vi "Change_RunInfo_V2.vi"(2 "error in (no error)":errorcluster, 3 "Run Data SubPanel in":T1) -> (0 "error out":errorcluster, 1 "Run Data SubPanel out":T1)   [LabVIEW 2019]
uses:
  Controls/DataBlockControl.ctl
panel:
  in  "Change Test Type":bool
  in  "Effective LET":bool
  in  "Update Board Number":bool
  in  "Update Ion":bool
  in  "Update DUT":bool
  in  "Update Path":bool
  out "Current Run Data":T1
  in  "Exit SubVI":bool
  in  "Run Data Input":T1
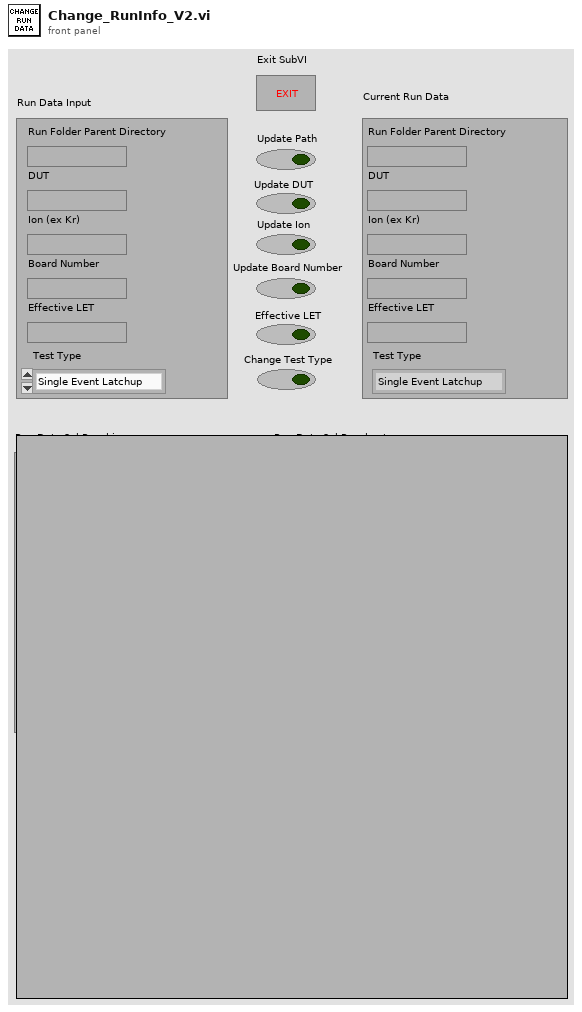
[diagram p1: front panel]
types:
  T1 = typedef "DataBlockControl.ctl" = cluster{"Run Folder Parent Directory":path, "DUT":string, "Ion (ex Kr)":string, "Board Number":string, "Effective LET":string, "Test Type":enum16{"Single Event Latchup", "Single Event Transient", "Single Event Upset"}}
  T2 = enum16{"Single Event Latchup", "Single Event Transient", "Single Event Upset"}
  T3 = cluster{"Run Folder Parent Directory":path, "DUT":string, "Ion (ex Kr)":string, "Board Number":string, "Effective LET":string, "Test Type":enum16{"Single Event Latchup", "Single Event Transient", "Single Event Upset"}}
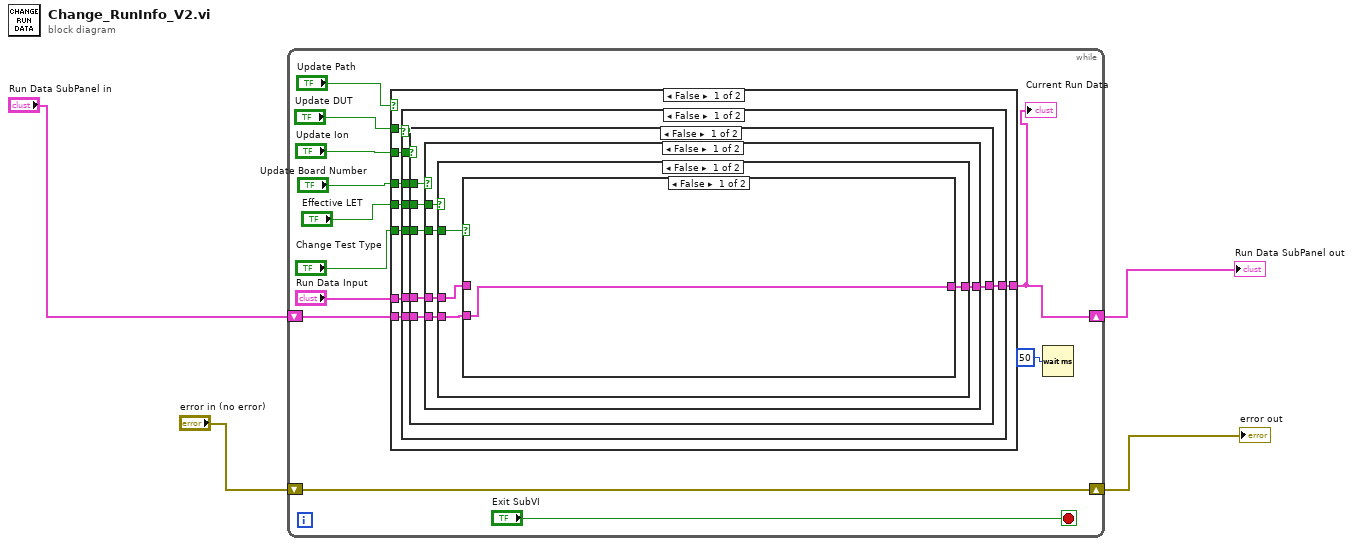
[diagram p0: block diagram]
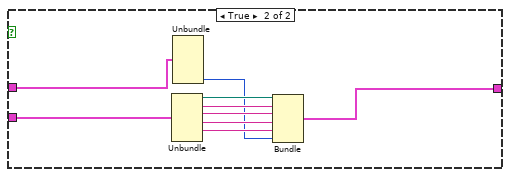
[diagram p2: hidden frame]
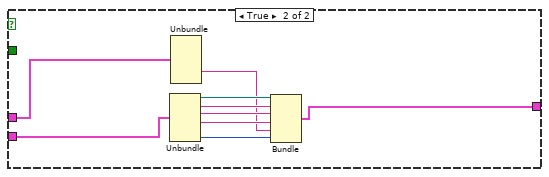
[diagram p3: hidden frame]
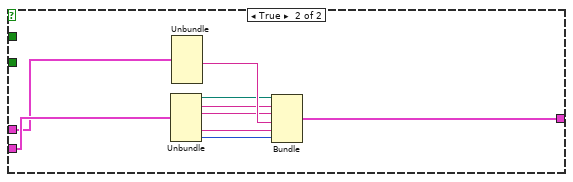
[diagram p4: hidden frame]
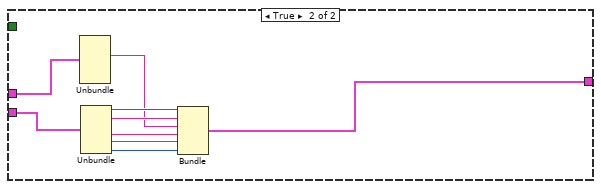
[diagram p5: hidden frame]
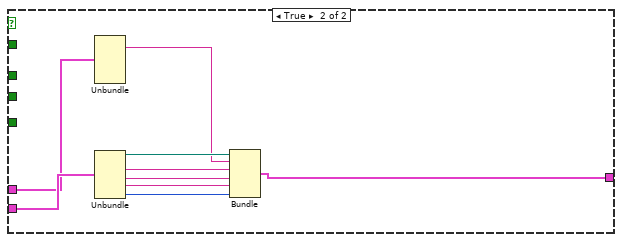
[diagram p6: hidden frame]
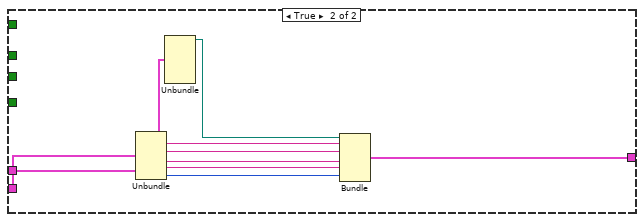
[diagram p7: hidden frame]
diagram:
  n1 = while {
    shift-right: [w6] -> w4
    shift-left: "Run Data SubPanel in" -> [w12]
    shift-right: [w14] -> w2
    shift-left: "error in (no error)" -> [w14]
    stop <- "Exit SubVI" stop-if-true
    n2 = case shown="False" "Update Path" {
      tunnel: w12 -> [w24 w101]
      tunnel: "Run Data Input" -> [w23 w94]
      tunnel: "Update DUT" -> [w22 _]
      tunnel: "Update Ion" -> [w21 _]
      tunnel: "Update Board Number" -> [w20 _]
      tunnel: "Effective LET" -> [w19 _]
      tunnel: [w18 w93] -> w6
      tunnel: "Change Test Type" -> [w17 _]
      frame False {
        n3 = case shown="False" w22 {
          tunnel: w24 -> [w31 w92]
          tunnel: w23 -> [w30 w91]
          tunnel: w21 -> [w29 _]
          tunnel: w20 -> [w28 _]
          tunnel: w19 -> [w27 _]
          tunnel: [w26 w84] -> w18
          tunnel: w17 -> [w25 _]
          frame False {
            n4 = case shown="False" w29 {
              tunnel: w31 -> [w37 w82]
              tunnel: w30 -> [w36 w83]
              tunnel: w28 -> [w35 _]
              tunnel: w27 -> [w34 _]
              tunnel: [w33 w75] -> w26
              tunnel: w25 -> [w32 _]
              frame False {
                n5 = case shown="False" w35 {
                  tunnel: w37 -> [w41 w68]
                  tunnel: w36 -> [w42 w67]
                  tunnel: w34 -> [w40 _]
                  tunnel: [w39 w66] -> w33
                  tunnel: w32 -> [w38 _]
                  frame False {
                    n6 = case shown="False" w40 {
                      tunnel: w42 -> [w46 w61]
                      tunnel: w41 -> [w45 w60]
                      tunnel: [w43 w58] -> w39
                      tunnel: w38 -> [w44 _]
                      frame False {
                        n7 = case shown="False" w44 {
                          tunnel: w46 -> [_ w52]
                          tunnel: w45 -> [w47 w51]
                          tunnel: [w47 w48] -> w43
                          frame False {
                          }
                          frame True {
                            n8 = Unbundle(w51) -> ("Run Folder Parent Directory"=w56:path, "DUT"=w55:string, "Ion (ex Kr)"=w54:string, "Board Number"=w53:string, "Effective LET"=w50:string)  [unwired: 1 out]
                            n9 = Unbundle(w52) -> ("Test Type"=w49:T2)  [unwired: 5 out]
                            n10 = Bundle("Run Folder Parent Directory"=w56, "DUT"=w55, "Ion (ex Kr)"=w54, "Board Number"=w53, "Effective LET"=w50, "Test Type"=w49) -> (w48:T3)  [unwired: 1 in]
                          }
                        }
                      }
                      frame True {
                        n11 = Unbundle(w60) -> ("Run Folder Parent Directory"=w65:path, "DUT"=w64:string, "Ion (ex Kr)"=w63:string, "Board Number"=w59:string, "Test Type"=w62:T2)  [unwired: 1 out]
                        n12 = Unbundle(w61) -> ("Effective LET"=w57:string)  [unwired: 5 out]
                        n13 = Bundle("Run Folder Parent Directory"=w65, "DUT"=w64, "Ion (ex Kr)"=w63, "Board Number"=w59, "Effective LET"=w57, "Test Type"=w62) -> (w58:T3)  [unwired: 1 in]
                      }
                    }
                  }
                  frame True {
                    n14 = Unbundle(w68) -> ("Run Folder Parent Directory"=w73:path, "DUT"=w72:string, "Ion (ex Kr)"=w71:string, "Effective LET"=w70:string, "Test Type"=w69:T2)  [unwired: 1 out]
                    n15 = Unbundle(w67) -> ("Board Number"=w74:string)  [unwired: 5 out]
                    n16 = Bundle("Run Folder Parent Directory"=w73, "DUT"=w72, "Ion (ex Kr)"=w71, "Board Number"=w74, "Effective LET"=w70, "Test Type"=w69) -> (w66:T3)  [unwired: 1 in]
                  }
                }
              }
              frame True {
                n17 = Unbundle(w83) -> ("Ion (ex Kr)"=w79:string)  [unwired: 5 out]
                n18 = Unbundle(w82) -> ("Run Folder Parent Directory"=w81:path, "DUT"=w80:string, "Board Number"=w78:string, "Effective LET"=w77:string, "Test Type"=w76:T2)  [unwired: 1 out]
                n19 = Bundle("Run Folder Parent Directory"=w81, "DUT"=w80, "Ion (ex Kr)"=w79, "Board Number"=w78, "Effective LET"=w77, "Test Type"=w76) -> (w75:T3)  [unwired: 1 in]
              }
            }
          }
          frame True {
            n20 = Unbundle(w91) -> ("DUT"=w89:string)  [unwired: 5 out]
            n21 = Unbundle(w92) -> ("Run Folder Parent Directory"=w90:path, "Ion (ex Kr)"=w88:string, "Board Number"=w87:string, "Effective LET"=w86:string, "Test Type"=w85:T2)  [unwired: 1 out]
            n22 = Bundle("Run Folder Parent Directory"=w90, "DUT"=w89, "Ion (ex Kr)"=w88, "Board Number"=w87, "Effective LET"=w86, "Test Type"=w85) -> (w84:T3)  [unwired: 1 in]
          }
        }
      }
      frame True {
        n23 = Unbundle(w101) -> ("DUT"=w99:string, "Ion (ex Kr)"=w98:string, "Board Number"=w97:string, "Effective LET"=w96:string, "Test Type"=w95:T2)  [unwired: 1 out]
        n24 = Unbundle(w94) -> ("Run Folder Parent Directory"=w100:path)  [unwired: 5 out]
        n25 = Bundle("Run Folder Parent Directory"=w100, "DUT"=w99, "Ion (ex Kr)"=w98, "Board Number"=w97, "Effective LET"=w96, "Test Type"=w95) -> (w93:T3)  [unwired: 1 in]
      }
    }
    "Current Run Data" <- w6
    n26 = Wait (ms)(milliseconds to wait=u32 50) -> ()  [unwired: 1 out]
  }
  "Run Data SubPanel out" <- w4
  "error out" <- w2
